vi "stopTest.vi"(8 "error in (no error)":errorcluster, 10 "model":refnum<class "Model.lvclass">, 11 "TestingState in":refnum<class "TestingState.lvclass">) -> (0 "error out":errorcluster, 2 "model 2":refnum<class "Model.lvclass">, 3 "TestingState out":refnum<class "TestingState.lvclass">)   [LabVIEW 2015, in "TestingState.lvclass"]
uses:
  TestingState.lvclass
  Model/Model/Model.lvclass
  Typedefs/StateSelector.ctl
  EnabledState/EnabledState.lvclass
  Typedefs/M1M3SSSTypedefs.lvlib
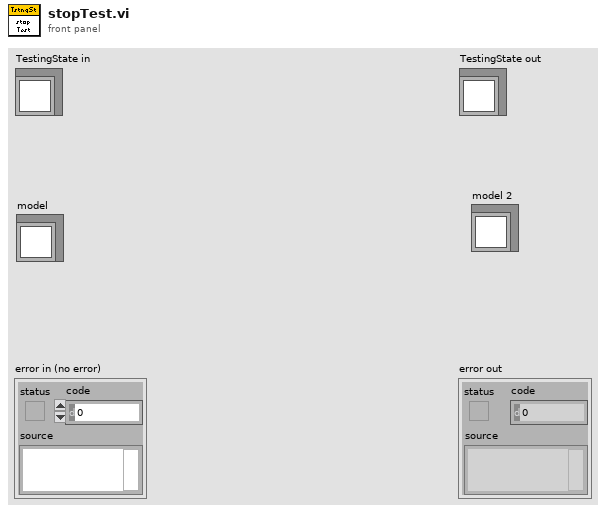
[diagram p1: front panel]
types:
  T1 = typedef "M1M3SSSTypedefs.lvlib/StateSelector.ctl" = enum16{"FaultState", "OffState", "RampingUpPressurePState", "RampingUpPressureSTState", "StandbyState", "StoppedState", "WaitingForSettledPState", "WaitingForSettledSTState"}
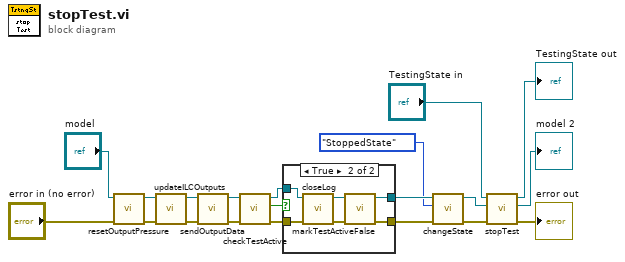
[diagram p0: block diagram]
diagram:
  n1 = call "resetOutputPressure.vi"("error in (no error)"="error in (no error)", "Model in"="model") -> ("error out"=w9:errorcluster, "Model out"=w11:refnum<class "Model.lvclass">)  [unwired: 8 in]
  n2 = call "updateILCOutputs.vi"("error in (no error)"=w9, "Model in"=w11) -> ("error out"=w8:errorcluster, "Model out"=w10:refnum<class "Model.lvclass">)  [unwired: 8 in]
  n3 = call "sendOutputData.vi"("error in (no error)"=w8, "Model in"=w10) -> ("error out"=w6:errorcluster, "Model out"=w7:refnum<class "Model.lvclass">)  [unwired: 8 in]
  n4 = call "checkTestActive.vi"("error in (no error)"=w6, "Model in"=w7) -> ("error out"=w12:errorcluster, "testActiveIsTrue"=w14:bool, "Model out"=w13:refnum<class "Model.lvclass">)  [unwired: 7 in]
  n5 = case shown="True" w14 {
    tunnel: [w22 w25] -> w16
    tunnel: [w21 w23] -> w15
    tunnel: w13 -> [w22 w28]
    tunnel: w12 -> [w21 w27]
    frame False {
    }
    frame True {
      n6 = call "closeLog.vi"("error in (no error)"=w27, "Model in"=w28) -> ("error out"=w24:errorcluster, "Model out"=w26:refnum<class "Model.lvclass">)  [unwired: 8 in]
      n7 = call "markTestActiveFalse.vi"("error in (no error)"=w24, "Model in"=w26) -> ("error out"=w23:errorcluster, "Model out"=w25:refnum<class "Model.lvclass">)  [unwired: 8 in]
    }
  }
  n8 = call "changeState.vi"("error in (no error)"=w15, "State:"=StateSelector."StoppedState", "Model in"=w16) -> ("error out"=w1:errorcluster, "Model out"=w4:refnum<class "Model.lvclass">)  [unwired: 7 in]
  n9 = call-parent "stopTest.vi"("error in (no error)"=w1, "model"=w4, "State in"="TestingState in") -> ("error out"=→"error out":errorcluster, "model 2"=→"model 2":refnum<class "Model.lvclass">, "State out"=→"TestingState out":refnum<class "TestingState.lvclass">)  [unwired: 6 in]
